vi "Get Copy Error Code Files.vi"(8 "error in (no error)":errorcluster, 11 "NI_AB_API_Application in":refnum<class "NI_AB_API_Application.lvclass">) -> (0 "error out":errorcluster, 2 "Copy error code files":bool, 3 "NI_AB_API_Application out":refnum<class "NI_AB_API_Application.lvclass">)   [LabVIEW 2020, in "NI_AB_API_Application.lvclass"]
uses:
  <vilib>/AppBuilder/AB_API/Application/NI_AB_API_Application.lvclass
  <vilib>/AppBuilder/AB_API/Application/NI_AB_API_Application.lvclass/NI_AB_API_Application.ctl
  <vilib>/AppBuilder/AB_Classes/Application/AB_Application.lvclass
  <vilib>/AppBuilder/AB_API/Build/NI_AB_API_Build.lvclass
  e:/builds/penguin/labview/branches/2020/dev/dist/vi.lib/AppBuilder/AB_API/Targetfile/NI_AB_API_Targetfile.lvclass
  e:/builds/penguin/labview/branches/2020/dev/dist/vi.lib/AppBuilder/AB_API/Build/NI_AB_API_Build.lvclass
  e:/builds/penguin/labview/branches/2020/dev/dist/vi.lib/AppBuilder/AB_API/Application/NI_AB_API_Application.lvclass
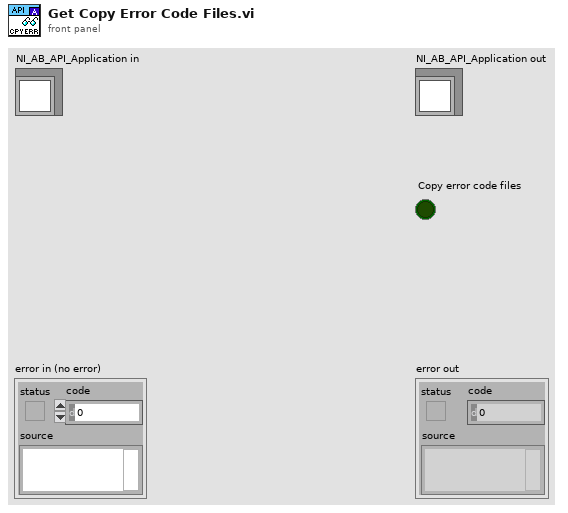
[diagram p1: front panel]
types:
  T1 = typedef "AB_Application.ctl" = cluster{"INI_path":path, "INI_itemID":string, "INI_GUID":string, "aliasPath":path, "aliasItemID":string, "aliasGUID":string, "waitDebugging":bool, "copyErrors":bool, "useFFRTE":bool, "includeHWConfig":bool, "showHWConfig":bool, "winsec.certificate":string, "winsec.timestamp":string, "winsec.description":string, "winsec.manifestItemID":string, "winsec.manifestPath":path, "web service itemIDs":string[], "Embedded Server Configuration":T2, "Server Type":enum32{"NI Web Server", "Application Web Server"}}
  T2 = typedef "AB_Embedded_Server_Configuration.ctl" = cluster{"HTTP enabled?":bool, "HTTP port":i32, "HTTPS enabled?":bool, "HTTPS port":i32, "SSL certificate file":path}
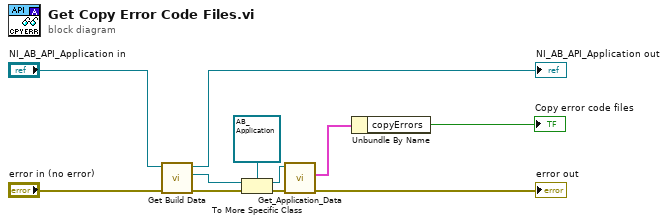
[diagram p0: block diagram]
diagram:
  n1 = call <vilib>:"Get Build Data.vi"("error in (no error)"="error in (no error)", "NI_AB_API_Build in"="NI_AB_API_Application in") -> ("error out"=w5:errorcluster, "AB_Build.lvclass"=w8:refnum<class "AB_Build.lvclass">, "NI_AB_API_Build out"=→"NI_AB_API_Application out":refnum<class "NI_AB_API_Application.lvclass">)  [unwired: 7 in]
  n2 = To More Specific Class(target class=refnum<class "AB_Application.lvclass"> refnum ("AB_Application in"), reference=w8, error in=w5) -> (specific class reference=w7:refnum<class "AB_Application.lvclass">, error out=w3:errorcluster)
  n3 = call <vilib>:"Get_Application_Data.vi"("error in (no error)"=w3, "AB_Application in"=w7) -> ("error out"=→"error out":errorcluster, "data"=w4:T1)  [unwired: 8 out]
  n4 = Unbundle By Name(w4) -> ("copyErrors"=→"Copy error code files":bool)
